vi "Compute Camera Frame 3D Coordinates.vi"(5 "cy height":dbl format="%.5f", 6 "f_px":dbl format="%.5f", 7 "cx width":dbl format="%.5f", 8 "World corner points (out)":dbl[][](array[numeric])=[[-3.25, -3.25, 0.0], [3.25, -3.25, 0.0], [3.25, 3.25, 0.0], [-3.25, 3.25, 0.0]], 9 "t Translation Vector":dbl[](array[numeric]), 10 "R Rotation Matrix":T1 format="%#_6f", 11 "Measured Points":dbl[][](array[numeric])) -> ()   [LabVIEW 2025]
uses:
  <vilib>/Analysis/Matrix/Datatypes/RealMatrix.ctl
  <vilib>/Analysis/5stat.llb/RMS (DBL).vi
  <vilib>/Analysis/baseanly.llb/Mean (DBL).vi
  <vilib>/Analysis/NI_AALBase.lvlib
  <vilib>/Analysis/NI_AALPro.lvlib
  <vilib>/Analysis/Matrix/NI_Matrix.lvlib
panel:
  out "RMS reprojection error":dbl format="%0.2f"
  out "Mean reprojection error":dbl format="%0.2f"
  out "Xc (in) (X,Y,Z)":dbl[][](array[numeric])
  out "reprojection error (px)":dbl[](array[numeric])
  out "v' (px)":dbl[](array[numeric])
  out "u' (px)":dbl[](array[numeric])
  out "p Array":dbl[][](array[numeric]) format="%#.6f"
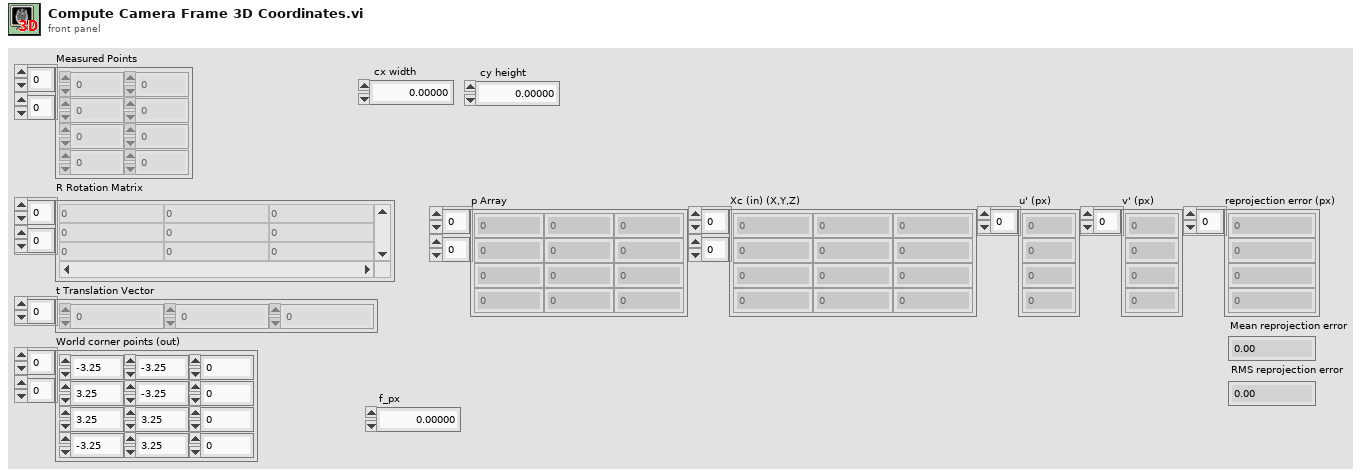
[diagram p1: front panel]
types:
  T1 = typedef "NI_Matrix.lvlib/RealMatrix.ctl" = dbl[][]
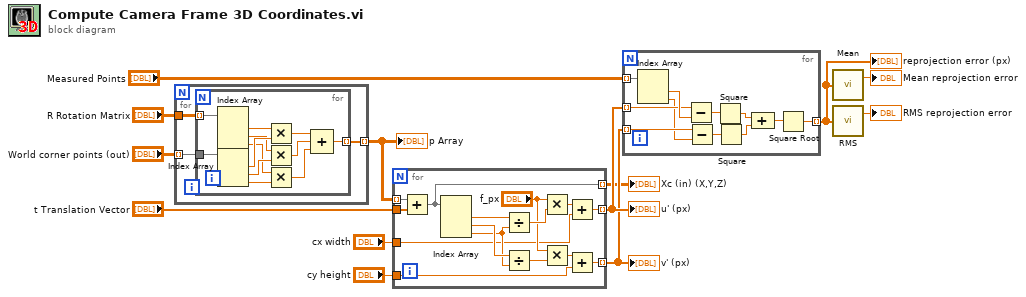
[diagram p0: block diagram]
diagram:
  n1 = for {
    tunnel: "World corner points (out)" -> [w16] mode=indexing
    tunnel: "R Rotation Matrix" -> [w15]
    tunnel: [w14] -> w11 mode=indexing
    n2 = for {
      tunnel: w15 -> [w28] mode=indexing
      tunnel: w16 -> [w27]
      tunnel: [w17] -> w14 mode=indexing
      n3 = Index Array(array=w28) -> (element #1=w26:dbl, element #2=w23:dbl, element #3=w21:dbl)  [unwired: 3 in]
      n4 = Index Array(array=w27) -> (element #1=w25:dbl, element #2=w22:dbl, element #3=w20:dbl)  [unwired: 3 in]
      n5 = Multiply(x=w26, y=w25) -> (x*y=w24:dbl)
      n6 = Multiply(x=w23, y=w22) -> (x*y=w19:dbl)
      n7 = Multiply(x=w21, y=w20) -> (x*y=w18:dbl)
      n8 = Compound Arithmetic op=ADD(w24, w19, w18) -> (w17:dbl)
    }
  }
  "p Array" <- w11
  n9 = for {
    tunnel: w11 -> [w43] mode=indexing
    tunnel: "t Translation Vector" -> [w42]
    tunnel: [w33] -> w8 mode=indexing
    tunnel: [w32] -> w7 mode=indexing
    tunnel: "cy height" -> [w31]
    tunnel: "cx width" -> [w30]
    tunnel: [w29] -> w4 mode=indexing
    n10 = Add(x=w43, y=w42) -> (x+y=w29:dbl[])
    n11 = Index Array(array=w29) -> (element #1=w41:dbl, element #2=w37:dbl, element #3=w36:dbl)  [unwired: 3 in]
    n12 = Divide(x=w41, y=w36) -> (x/y=w40:dbl)
    n13 = Divide(x=w37, y=w36) -> (x/y=w35:dbl)
    n14 = Multiply(x="f_px", y=w40) -> (x*y=w39:dbl)
    n15 = Multiply(x="f_px", y=w35) -> (x*y=w34:dbl)
    n16 = Add(x=w39, y=w30) -> (x+y=w33:dbl)
    n17 = Add(x=w34, y=w31) -> (x+y=w32:dbl)
  }
  "u' (px)" <- w8
  "v' (px)" <- w7
  "Xc (in) (X,Y,Z)" <- w4
  n18 = for {
    tunnel: "Measured Points" -> [w54] mode=indexing
    tunnel: w8 -> [w52] mode=indexing
    tunnel: w7 -> [w51] mode=indexing
    tunnel: [w45] -> w3 mode=indexing
    n19 = Index Array(array=w54) -> (element #1=w53:dbl, element #2=w50:dbl)  [unwired: 2 in]
    n20 = Subtract(x=w52, y=w53) -> (x-y=w49:dbl)
    n21 = Subtract(x=w51, y=w50) -> (x-y=w44:dbl)
    n22 = Square(x=w49) -> (x^2=w48:dbl)
    n23 = Square(x=w44) -> (x^2=w47:dbl)
    n24 = Compound Arithmetic op=ADD(w48, w47) -> (w46:dbl)
    n25 = Square Root(x=w46) -> (sqrt(x)=w45:dbl)
  }
  "reprojection error (px)" <- w3
  n26 = call-poly <vilib>:"Mean.vi"("X"=w3) -> ("mean"=→"Mean reprojection error":dbl)  [unwired: 1 out]
  n27 = call-poly <vilib>:"RMS.vi"("X"=w3) -> ("rms value"=→"RMS reprojection error":dbl)  [unwired: 1 out]
